vi "XY Plot with Error Bars.vi"(0 "Data In":T4, 2 "Display State In":T2, 3 "Container State":T3) -> (6 "Data Out":T4, 7 "Display State Out":T2, 8 "Action":T1)   [LabVIEW 2012, in "XY Plot with Error Bars.xctl"]
uses:
  XY Plot with Error Bars.xctl
  Data.ctl
  <vilib>/_xctls/Container State.ctl
  State.ctl
  <vilib>/_xctls/Action.ctl
  <vilib>/_xctls/XControlSupport.lvlib
panel:
  out "Plot":cluster{"Data Out":dbl[], "Data Out":dbl[]}[](graph)
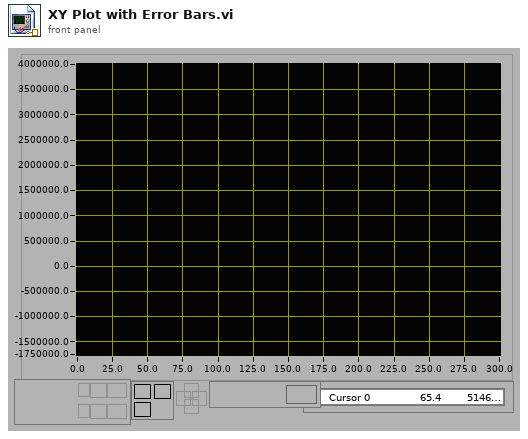
[diagram p1: front panel]
types:
  T1 = typedef "XControlSupport.lvlib/Action.ctl" = cluster{"Data Changed?":bool, "State Changed?":bool, "Action Name":string}
  T2 = typedef "XY Plot with Error Bars.xctl/State.ctl" = cluster{"XCTLRefs":refnum<vi>[], "Delta X":dbl[], "Delta Y":dbl[]}
  T3 = typedef "XControlSupport.lvlib/Container State.ctl" = cluster{"Indicator?":bool, "Run Mode?":bool, " Refnum":refnum<vi>}
  T4 = typedef "XY Plot with Error Bars.xctl/Data.ctl" = cluster{"X":dbl[], "Y":dbl[]}
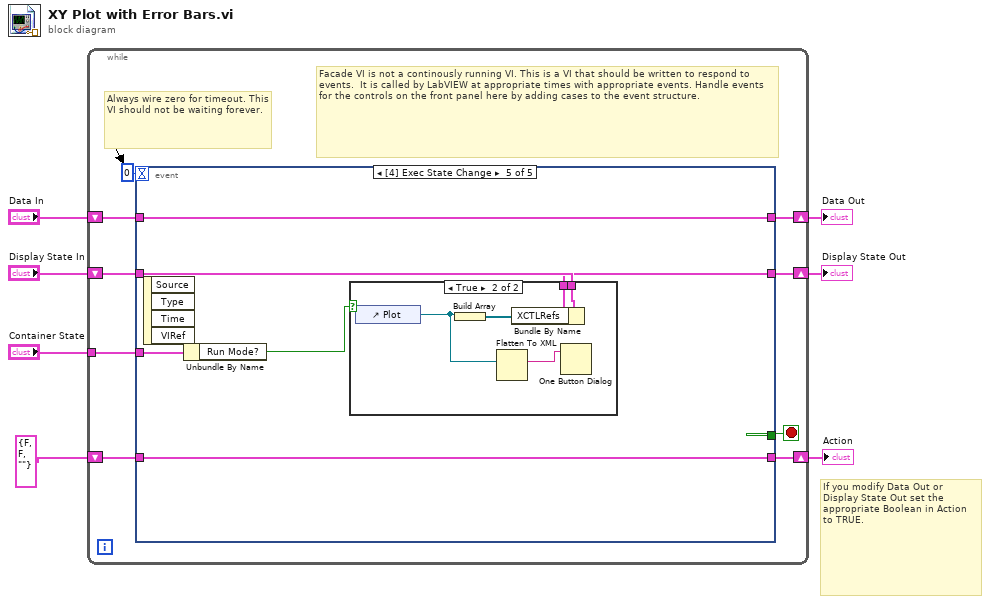
[diagram p0: block diagram]
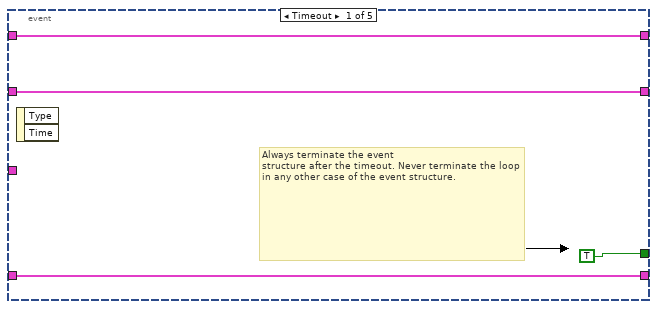
[diagram p2: hidden frame]
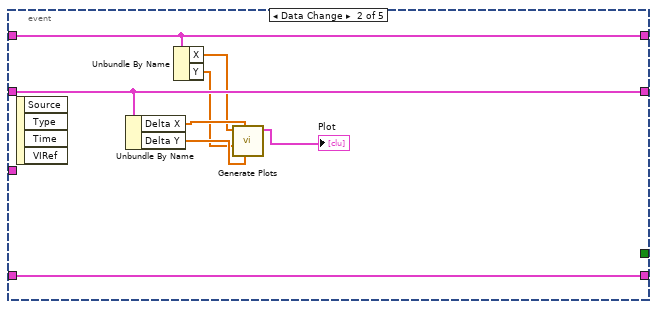
[diagram p3: hidden frame]
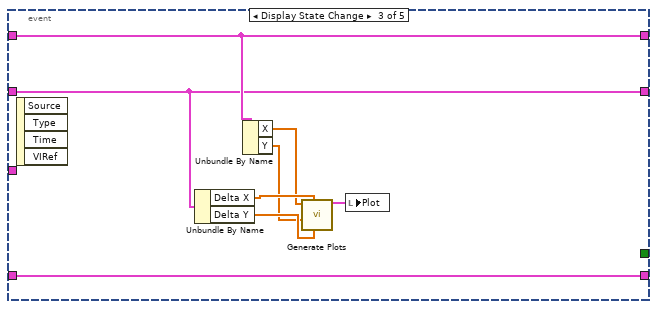
[diagram p4: hidden frame]
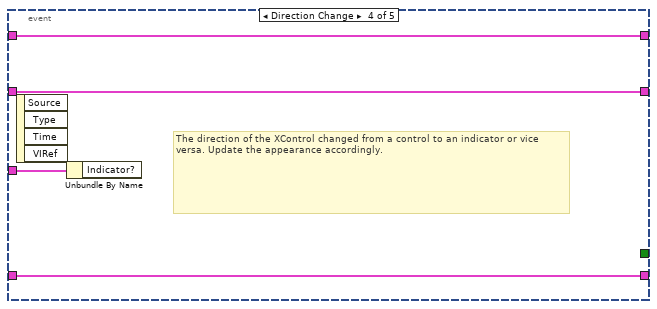
[diagram p5: hidden frame]
diagram:
  # "If you modify Data Out or\nDisplay State Out set the\nappropriate Boolean in Action\nto TRUE."
  n1 = while {
    shift-right: [w15] -> w4
    shift-left: "Display State In" -> [w16]
    tunnel: "Container State" -> [w12]
    shift-right: [w10] -> w7
    shift-left: "Data In" -> [w11]
    shift-right: [w8] -> w2
    shift-left: T1 {"Data Changed?"=FALSE, "State Changed?"=FALSE, "Action Name"=""} ("Action") -> [w9]
    stop <- w14 stop-if-true
    # "Facade VI is not a continously running VI. This is a VI that should be written to respond to events.  It is called by LabVIEW at appropriate times with appropriate events. Handle events for the controls on the front panel here by adding cases to the event structure."
    # "Always wire zero for timeout. This\nVI should not be waiting forever."
    n2 = event shown="[4] Exec State Change" {
      selector: _ -> [_ _ _ _ _]
      dyn-events: _ -> [_ _ _ _ _]
      timeout: 0 -> [_ _ _ _ _]
      tunnel: w16 -> [w18 w27 w30 w39 w43]
      tunnel: [w18 w27 w30 w39 w42] -> w15
      tunnel: [TRUE _ _ _ _] -> w14
      tunnel: w12 -> [_ _ _ w40 w46]
      tunnel: w11 -> [w17 w24 w31 w38 w45]
      tunnel: [w17 w24 w31 w38 w45] -> w10
      tunnel: [w19 w28 w36 w37 w44] -> w8
      tunnel: w9 -> [w19 w28 w36 w37 w44]
      event Timeout {
        # "Always terminate the event\nstructure after the timeout. Never terminate the loop in any other case of the event structure."
        n3 = event-data() -> ()  [unwired: 3 out]
      }
      event Data Change {
        n4 = event-data() -> ()  [unwired: 5 out]
        n5 = Unbundle By Name(w27) -> ("Delta X"=w26:dbl[], "Delta Y"=w25:dbl[])
        n6 = Unbundle By Name(w24) -> ("X"=w22:dbl[], "Y"=w23:dbl[])
        n7 = call "Generate Plots.vi"("Y Errors"=w25, "X Errors"=w26, "Y Data"=w23, "X Data"=w22) -> ("Plot Data"=→"Plot":cluster{"X Data":dbl[], "Y Data":dbl[]}[])  [unwired: 7 out]
      }
      event Display State Change {
        n8 = event-data() -> ()  [unwired: 5 out]
        n9 = Unbundle By Name(w30) -> ("Delta X"=w35:dbl[], "Delta Y"=w34:dbl[])
        n10 = Unbundle By Name(w31) -> ("X"=w32:dbl[], "Y"=w33:dbl[])
        n11 = call "Generate Plots.vi"("Y Errors"=w34, "X Errors"=w35, "Y Data"=w33, "X Data"=w32) -> ("Plot Data"=w29:cluster{"X Data":dbl[], "Y Data":dbl[]}[])  [unwired: 7 out]
        n12 = local write "Plot"(w29) -> ()
      }
      event Direction Change {
        # "The direction of the XControl changed from a control to an indicator or vice versa. Update the appearance accordingly."
        n13 = event-data() -> ()  [unwired: 5 out]
        n14 = Unbundle By Name(w40) -> ()  [unwired: 1 out]
      }
      event Exec State Change {
        n15 = event-data() -> ()  [unwired: 5 out]
        n16 = Unbundle By Name(w46) -> ("Run Mode?"=w41:bool)
        n17 = case shown="True" w41 {
          tunnel: w43 -> [w47 w52]
          tunnel: [w47 w51] -> w42
          frame False {
          }
          frame True {
            n18 = control-ref of="Plot"() -> (w49:refnum<vi>)
            n19 = Build Array(w49) -> (w50:refnum<vi>[])
            n20 = Flatten To XML(anything=w49) -> (xml string=w48:string)
            n21 = Bundle By Name(cluster=w52, "XCTLRefs"=w50) -> (w51:T2)
            n22 = One Button Dialog(message=w48) -> ()  [unwired: 2 out]
          }
        }
      }
    }
  }
  "Display State Out" <- w4
  "Data Out" <- w7
  "Action" <- w2
